vi "ABB heat rdgs.vi"(6 "Run Time":dbl, 8 "Readings in":dbl[][](array[numeric]), 9 "Addnl temps":dbl[](array[numeric]), 10 "temperatures":dbl[](array[numeric]), 11 "power":dbl[](array[numeric])) -> (0 "Readings out":dbl[][](array[numeric]), 2 "Temperature trend":cluster{dbl[], dbl[]}[](array[cluster]), 4 "dT":dbl, 5 "rise rate":dbl)   [LabVIEW 2017]
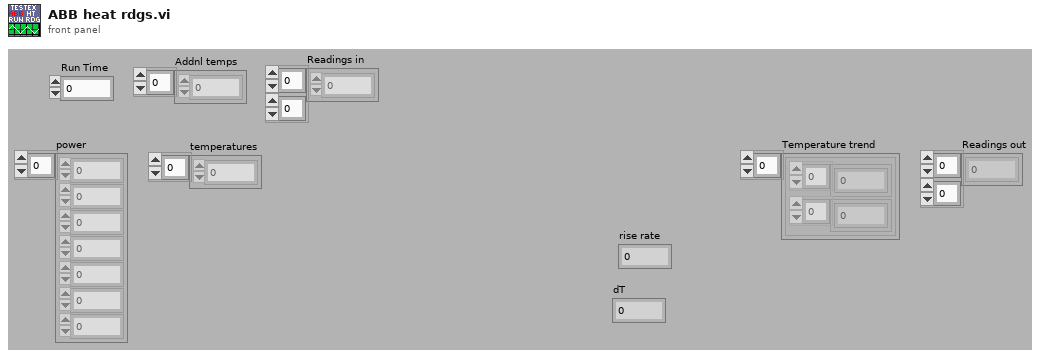
[diagram p1: front panel]
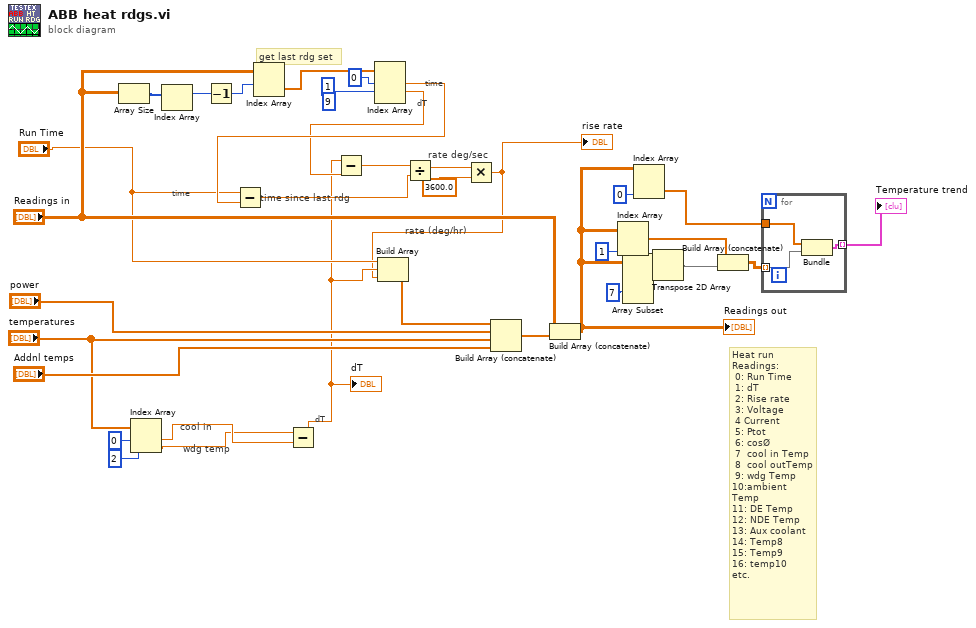
[diagram p0: block diagram]
diagram:
  (unwired) 9 ("index")
  # "rate (deg/hr)"
  # "rate deg/sec"
  # "dT"
  # "time since last rdg"
  # "time"
  # "time"
  # "Heat run Readings:\n 0: Run Time\n 1: dT\n 2: Rise rate\n 3: Voltage\n 4 Current\n 5: Ptot\n 6: cosØ\n 7  cool in Temp\n 8  cool outTemp\n 9: wdg Temp\n10:ambient Temp\n11: DE Temp\n12: NDE Temp\n13: Aux coolant\n14: Temp8\n15: Temp9\n16: temp10\netc."
  # "get last rdg set"
  # "dT"
  # "cool in"
  # "wdg temp"
  n1 = Array Size(array="Readings in") -> (size(s)=w22:i32[])
  n2 = Index Array(array="temperatures", index #1=0 ("index"), index #2=2 ("index")) -> (element #1=w24:dbl, element #2=w16:dbl)
  n3 = Index Array(array=w22) -> (element=w21:i32)  [unwired: 1 in]
  n4 = Decrement(x=w21) -> (x-1=w20:i32)
  n5 = Index Array(array="Readings in", index (row)=w20) -> (element=w19:dbl[])  [unwired: 1 in]
  n6 = Subtract(x=w16, y=w24) -> (x-y=w9:dbl)
  "dT" <- w9
  n7 = Index Array ("Run time")(array=w19, index #1=0 ("index"), index #2=1 ("index")) -> (element #1=w14:dbl, element #2=w13:dbl)  [unwired: 1 in, 1 out]
  n8 = Subtract(x="Run Time", y=w14) -> (x-y=w11:dbl)
  n9 = Subtract(x=w9, y=w13) -> (x-y=w12:dbl)
  n10 = Divide(x=w12, y=w11) -> (x/y=w8:dbl)
  n11 = Multiply(x=w8, y=3600.0) -> (x*y=w6:dbl)
  "rise rate" <- w6
  n12 = Build Array("Run Time", w9, w6) -> (w5:dbl[])
  n13 = Build Array (concatenate)(w5, "power", "temperatures", "Addnl temps") -> (w28:dbl[])
  n14 = Build Array (concatenate)("Readings in", w28) -> (w4:dbl[][])
  "Readings out" <- w4
  n15 = Index Array(array=w4, index (col)=1 ("disabled index (col)")) -> (element=w1:dbl[])  [unwired: 1 in]
  n16 = Array Subset(array=w4, index (col)=7 ("index")) -> (w32:dbl[][])  [unwired: 3 in]
  n17 = Index Array(array=w4, index (col)=0 ("disabled index (col)")) -> (element=w30:dbl[])  [unwired: 1 in]
  n18 = Transpose 2D Array(2D array=w32) -> (transposed array=w34:dbl[][])
  n19 = Build Array (concatenate)(w1, w34) -> (w2:dbl[][])
  n20 = for {
    tunnel: w30 -> [w38]
    tunnel: w2 -> [w36] mode=indexing
    tunnel: [w37] -> w33 mode=indexing
    n21 = Bundle(w38, w36) -> (w37:cluster{dbl[], dbl[]})  [unwired: 1 in]
  }
  "Temperature trend" <- w33
